vi "test3.vi"() -> ()   [LabVIEW 2010]
uses:
  Q - not nan -- real.vi
panel:
  out "in range?":bool=TRUE
  out "number in range":dbl
  in  "upper":dbl=inf
  in  "lower":dbl=-inf
  in  "number":dbl=11.0
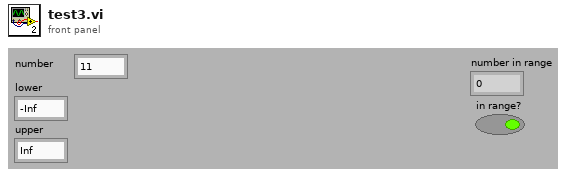
[diagram p1: front panel]
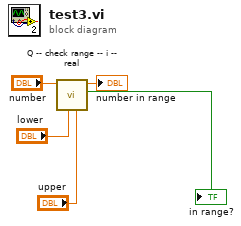
[diagram p0: block diagram]
diagram:
  n1 = call "Q -- check range -- i -- real.vi"("upper"="upper", "lower"="lower", "number"="number") -> ("in range?"=→"in range?":bool, "number in range"=→"number in range":dbl)  [unwired: 6 in, 1 out]
